vi "Set Experiment Body.vi"(7 "append (false)":bool, 8 "error in (no error)":errorcluster, 9 "body":string, 10 "experiment id":u32, 11 "eLab in":refnum<class "PL eLabFTW Client.lvclass">) -> (0 "error out":errorcluster, 3 "eLab out":refnum<class "PL eLabFTW Client.lvclass">)   [LabVIEW 2015, in "PL eLabFTW Client.lvclass"]
doc: "Sets or appends to experiment body."
uses:
  PL eLabFTW Client.lvclass
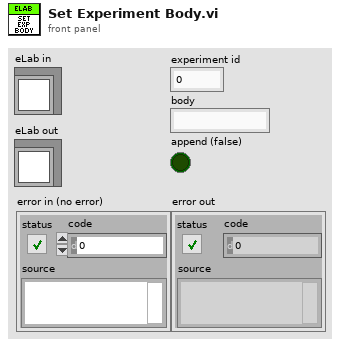
[diagram p1: front panel]
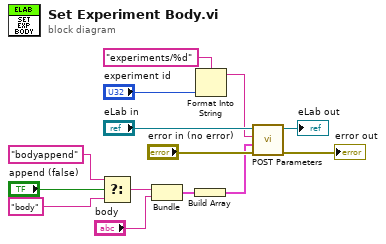
[diagram p0: block diagram]
diagram:
  n1 = Select(t="bodyappend" ("format string"), s="append (false)", f="body" ("format string")) -> (s? t:f=w5:string)
  n2 = Bundle("format string"=w5, "body"="body") -> (w4:cluster{"format string":string, "body":string})  [unwired: 1 in]
  n3 = Build Array(w4) -> (w1:cluster{"format string":string, "body":string}[])
  n4 = Format Into String(format string="experiments/%d", "experiment id") -> (resulting string=w8:string)  [unwired: 2 in, 1 out]
  n5 = call "POST Parameters.vi"("error in (no error)"="error in (no error)", "parameters"=w1, "relative URL"=w8, "eLab in"="eLab in") -> ("error out"=→"error out":errorcluster, "eLab out"=→"eLab out":refnum<class "PL eLabFTW Client.lvclass">)  [unwired: 5 in, 1 out]
